vi "ReportEnd_A131258.vi"(6 "文件重命名":bool, 8 "error in (no error)":errorcluster caption="错误输入（无错误）", 10 "文件名称":string, 11 "report in":refnum<class "NI_report.lvclass"> caption="报表输入") -> (0 "error out":errorcluster caption="错误输出")   [LabVIEW 2020]
uses:
  <vilib>/Utility/NIReport.llb/NI_report.lvclass
  Database/Global1.vi
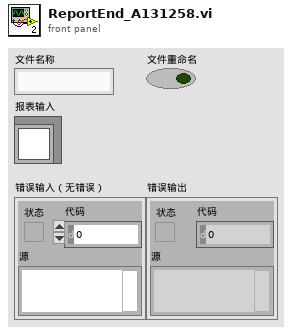
[diagram p1: front panel]
types:
  T1 = cluster{"Italic":enum16{"Italic Unchanged", "Italic On", "Italic Off"}, "Strike Through":enum16{"Strike Through Unchanged", "Strike Through On", "Strike Through Off"}, "Underline":enum16{"Underline Unchanged", "Underline On", "Underline Off"}, "Bold":enum16{"Bold Unchanged", "Bold On", "Bold Off"}}
  T2 = cluster{"Charset (-1)":i16, "Weight (-1)":i16, "Name":string, "Size":string}
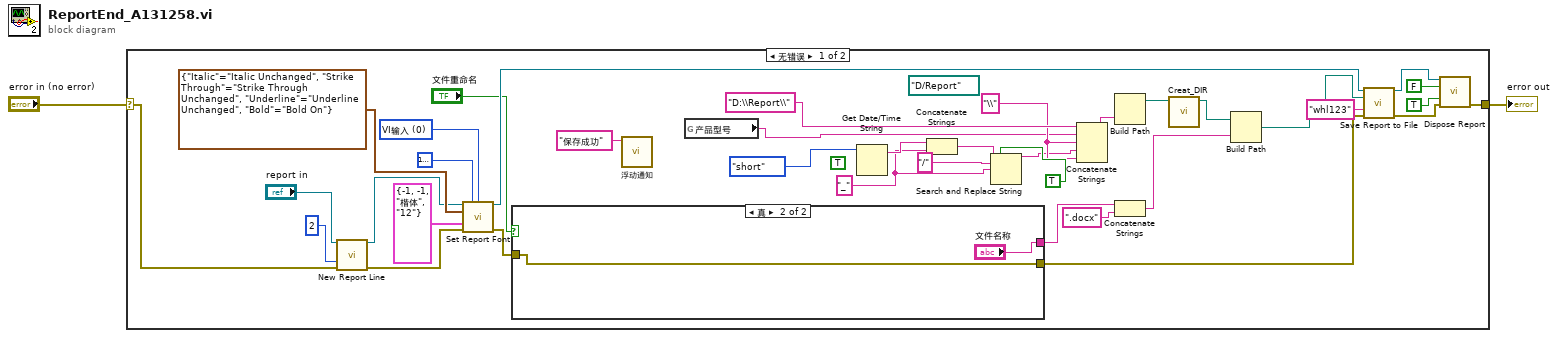
[diagram p0: block diagram]
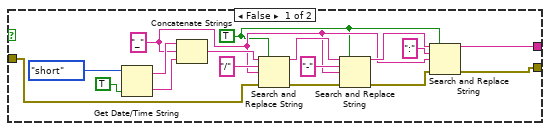
[diagram p2: hidden frame]
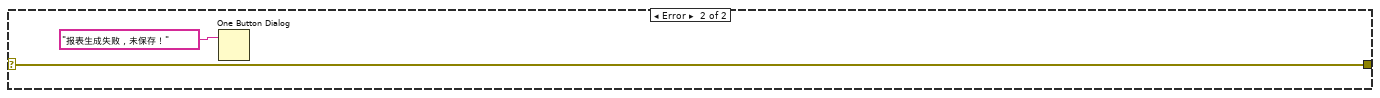
[diagram p3: hidden frame]
diagram:
  n1 = case shown="无错误" "error in (no error)" {
    selector: "error in (no error)" -> [w24 w60]
    tunnel: [w23 w60] -> w1
    frame No Error {
      w7 = "\\" ("替换字符串(\"\")")
      (unwired) TRUE ("需要秒？(F)")
      w10 = "_" ("替换字符串(\"\")")
      (unwired) path "D:/Report" ("report file path")
      w34 = u16 0 items=["VI输入", "字体对话框"] ("font settings source")
      n2 = call-dynamic "New Report Line.vi"("report in"="report in", "number of lines (1)"=2, "error in (no error)"=w24) -> ("report out"=w31:refnum<class "NI_report.lvclass">, "error out"=w30:errorcluster)  [unwired: 11 in]
      n3 = call-dynamic "Set Report Font.vi"("report in"=w31, "text color (unchanged)"=u32 16777224, "font settings source (VI Inputs)"=w34, "text options"=T1 {"Italic"=enum."Italic Unchanged", "Strike Through"=enum."Strike Through Unchanged", "Underline"=enum."Underline Unchanged", "Bold"=enum."Bold On"}, "font settings"=T2 {"Charset (-1)"=-1, "Weight (-1)"=-1, "Name"="楷体", "Size"="12"}, "error in (no error)"=w30) -> ("report out"=w27:refnum<class "NI_report.lvclass">, "error out"=w26:errorcluster)  [unwired: 7 in, 1 out]
      n4 = case shown="真" "文件重命名" {
        tunnel: [w51 "文件名称"] -> w21
        tunnel: w26 -> [w43 w57]
        tunnel: [w40 w57] -> w25
        frame False {
          w45 = TRUE ("替换全部？(F)")
          w46 = "_" ("替换字符串(\"\")")
          n5 = Get Date/Time String(date format (0)=enum16{"short", "long", "abbreviated"}."short" ("日期格式(0)"), want seconds? (F)=TRUE ("需要秒？(F)")) -> (date string=w56:string, time string=w52:string)  [unwired: 1 in]
          n6 = Concatenate Strings(w56, w46, w52) -> (w49:string)
          n7 = Search and Replace String(replace all?=w45, input string=w49, search string="/" ("搜索字符串"), replace string=w46, error in=w43) -> (result string=w48:string, error out=w42:errorcluster)  [unwired: 3 in, 2 out]
          n8 = Search and Replace String(replace all?=w45, input string=w48, search string="-" ("搜索字符串"), replace string=w46, error in=w42) -> (result string=w54:string, error out=w41:errorcluster)  [unwired: 3 in, 2 out]
          n9 = Search and Replace String(replace all?=w45, input string=w54, search string=":" ("搜索字符串"), replace string=w46, error in=w41) -> (result string=w51:string, error out=w40:errorcluster)  [unwired: 3 in, 2 out]
        }
        frame True {
        }
      }
      n10 = call "浮动通知.vi"("通知内容"="保存成功") -> ()  [unwired: 11 in]
      n11 = global read "Global1.vi" "产品型号"() -> (w5:string)
      n12 = Get Date/Time String(date format (0)=enum16{"short", "long", "abbreviated"}."short" ("日期格式(0)")) -> (date string=w14:string)  [unwired: 2 in, 1 out]
      n13 = Concatenate Strings(w14, w10) -> (w13:string)
      n14 = Search and Replace String(replace all?=TRUE ("替换全部？(F)"), input string=w13, search string="/" ("搜索字符串"), replace string=w10) -> (result string=w6:string)  [unwired: 4 in, 3 out]
      n15 = Concatenate Strings("D:\\Report\\", w5, w7, w6, w7) -> (w8:string)
      n16 = Build Path(name or relative path=w8) -> (appended path=w19:path)  [unwired: 1 in]
      n17 = Concatenate Strings(w21, ".docx" ("字符串")) -> (w17:string)
      n18 = call "Creat_DIR.vi"("path"=w19) -> ("created path"=w18:path)  [unwired: 10 in]
      n19 = Build Path(base path=w18, name or relative path=w17) -> (appended path=w16:path)
      n20 = call-dynamic "Save Report to File.vi"("report in"=w27, "report file path"=w16, "password (\"\")"="whl123" ("password (\"\")"), "error in (no error)"=w25) -> ("report out"=w39:refnum<class "NI_report.lvclass">, "error out"=w38:errorcluster)  [unwired: 10 in]
      n21 = call-dynamic "Dispose Report.vi"("report in"=w39, "wait until printing completed? (T)"=FALSE, "save changes? (F)"=TRUE, "error in (no error)"=w38) -> ("error out"=w23:errorcluster)  [unwired: 11 in]
    }
    frame Error {
      n22 = One Button Dialog(message="报表生成失败，未保存！" ("消息")) -> ()  [unwired: 1 in, 1 out]
    }
  }
  "error out" <- w1
